vi "SUM OF SQUARES.vi"() -> ()   [LabVIEW 2018]
panel:
  out "A^2+B^2":dbl(knob) scale=0.0..100.0
  in  "B":dbl
  in  "A":dbl
  out "A^2+B^2":dbl
  # "Sum of Squares"
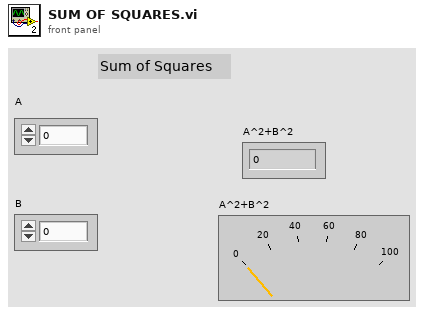
[diagram p1: front panel]
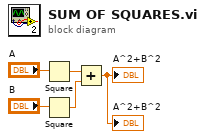
[diagram p0: block diagram]
diagram:
  n1 = Square(x="A") -> (x^2=w5:dbl)
  n2 = Square(x="B") -> (x^2=w4:dbl)
  n3 = Add(x=w5, y=w4) -> (x+y=→"A^2+B^2" →"A^2+B^2":dbl)
